vi "Write Homing.vi"(8 "error in (no error)":errorcluster, 10 "Homing":variant, 11 "FW Arduino Control in":refnum<class "FW Arduino Control.lvclass">) -> (0 "error out":errorcluster, 3 "FW Arduino Control out":refnum<class "FW Arduino Control.lvclass">)   [LabVIEW 2024, in "FW Arduino Control.lvclass"]
uses:
  FW Arduino Control.lvclass
  Filter Wheel Arduino Homing cluster.ctl
  FW Arduino Control.lvclass/FW Arduino Control.ctl
  Filter Wheel Object/Filter Wheel.lvclass
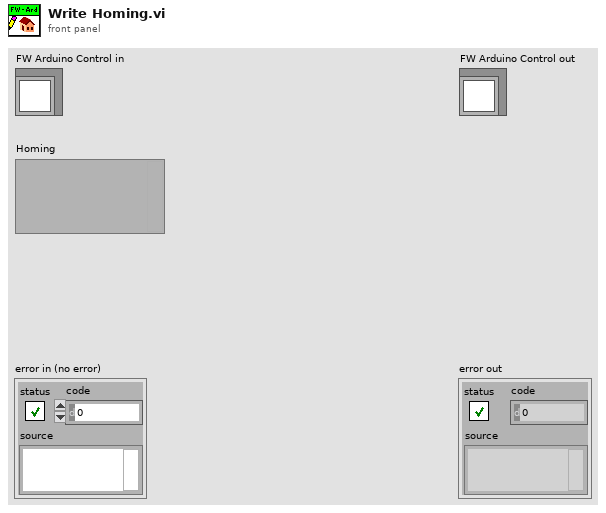
[diagram p1: front panel]
types:
  T1 = typedef "Filter Wheel Arduino Homing cluster.ctl" = cluster{"Direction":bool, "Speed":i32, "Accel":i32, "Error Cnts":i32, "Homing Delta":i32}
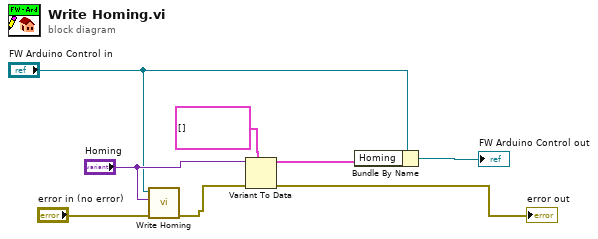
[diagram p0: block diagram]
diagram:
  n1 = call-parent "Write Homing.vi"("error in (no error)"="error in (no error)", "Homing"="Homing", "Filter Wheel in"="FW Arduino Control in") -> ("error out"=w6:errorcluster)  [unwired: 7 in, 1 out]
  n2 = Variant To Data(error in=w6, type=T1[] [], Variant="Homing") -> (data=w2:T1[], error out=→"error out":errorcluster)
  n3 = Bundle By Name(cluster="FW Arduino Control in", "Homing"=w2) -> (→"FW Arduino Control out":refnum<class "FW Arduino Control.lvclass">)
